vi "test_EnumerateComputeNodes_StopDiscoveryService_EnumerateComputeNodesWorkWithoutError.vi"(8 "error in":errorcluster) -> (0 "error out":errorcluster, 2 "result":string, 3 "pass":bool)   [LabVIEW 2021, in "MeasurementServerTests.lvlib" / "Discovery Tests.lvlib"]
uses:
  Discovery Tests.lvlib
  gRPC/Generated APIs/ni/measurementlink/discovery/v1/RPC Messages/ni_measurementlink_discovery_v1_EnumerateComputeNodesRequest.ctl
  MeasurementServerTests.lvlib
  Runtime/Clients/Discovery V1/NI Discovery V1 Client.lvlib
  gRPC/Generated APIs/ni/measurementlink/discovery/v1/ni.measurementlink.discovery.v1.api.lvlib
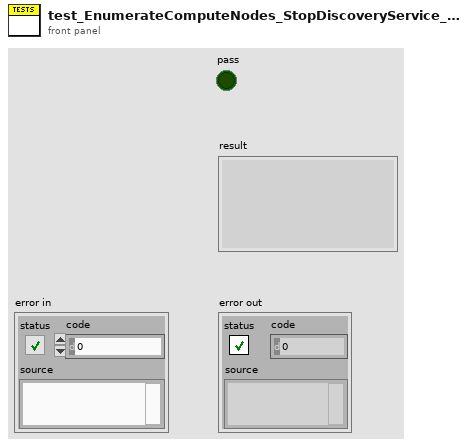
[diagram p1: front panel]
types:
  T1 = typedef "ni.measurementlink.discovery.v1.api.lvlib/ni_measurementlink_discovery_v1_EnumerateComputeNodesRequest.ctl" = cluster{"void":string}
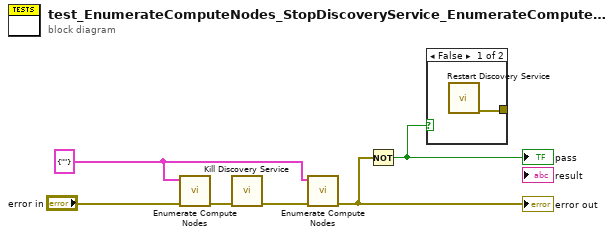
[diagram p0: block diagram]
diagram:
  w2 = T1 {"void"=""} ("request data")
  n1 = call "Enumerate Compute Nodes.vi"("error in"="error in", "request data"=w2) -> ("error out"=w3:errorcluster)  [unwired: 8 in, 1 out]
  n2 = call "Kill Discovery Service.vi"("error in"=w3) -> ("error out"=w5:errorcluster)  [unwired: 10 in]
  n3 = call "Enumerate Compute Nodes.vi"("error in"=w5, "request data"=w2) -> ("error out"=w6:errorcluster)  [unwired: 8 in, 1 out]
  "error out" <- w6
  n4 = Not(x=w6) -> (.not. x?=w1:bool)
  "pass" <- w1
  n5 = case shown="False" w1 {
    tunnel: [w7 _] -> _
    frame False {
      n6 = call "Restart Discovery Service.vi"() -> ("error out"=w7:errorcluster)  [unwired: 11 in]
    }
    frame True {
    }
  }
